vi "dummy1.vi"() -> ()   [LabVIEW 2017]
panel:
  in  "_DUMMY VI_":string[][](table)
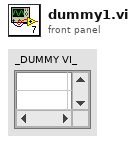
[diagram p1: front panel]
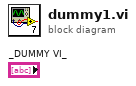
[diagram p0: block diagram]
diagram:
